vi "Write load inventory.vi"(8 "error in (no error)":errorcluster, 10 "load inventory":cluster{"String":string, "value":u32, bool}[][](array[cluster]), 11 "User Interface in":refnum<class "User Interface.lvclass">) -> (0 "error out":errorcluster, 3 "User Interface out":refnum<class "User Interface.lvclass">)   [LabVIEW 2020, in "User Interface.lvlib" / "User Interface.lvclass"]
uses:
  User Interface.lvclass
  User Interface.lvclass/User Interface.ctl
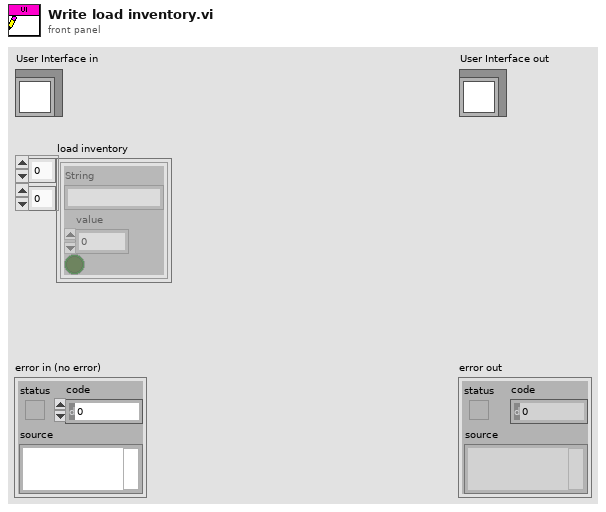
[diagram p1: front panel]
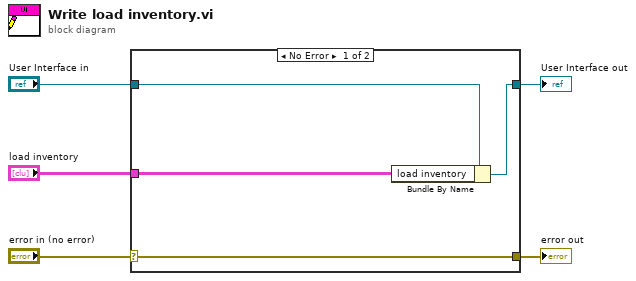
[diagram p0: block diagram]
diagram:
  n1 = case shown="No Error" "error in (no error)" {
    selector: "error in (no error)" -> [w9 w10]
    tunnel: [w9 w10] -> w4
    tunnel: [w7 w11] -> w2
    tunnel: "User Interface in" -> [w8 w11]
    tunnel: "load inventory" -> [w6 _]
    frame No Error {
      n2 = Bundle By Name(cluster=w8, "load inventory"=w6) -> (w7:refnum<class "User Interface.lvclass">)
    }
    frame Error {
    }
  }
  "error out" <- w4
  "User Interface out" <- w2
